vi "FipsAdjacent.vi"() -> (11 "Fips":i32[](array[numeric]))   [LabVIEW 2017] (continued)
41067\t\"Tillamook County, OR\"\t41057\n\"Washington County, OR\"\t41067\t\"Washington County, OR\"\t41067\n\"Washington County, OR\"\t41067\t\"Yamhill County, OR\"\t41071\n\"Wheeler County, OR\"\t41069\t\"Crook County, OR\"\t41013\n\"Wheeler County, OR\"\t41069\t\"Gilliam County, OR\"\t41021\n\"Wheeler County, OR\"\t41069\t\"Grant County, OR\"\t41023\n\"Wheeler County, OR\"\t41069\t\"Jefferson County, OR\"\t41031\n\"Wheeler County, OR\"\t41069\t\"Morrow County, OR\"\t41049\n\"Wheeler County, OR\"\t41069\t\"Wasco County, OR\"\t41065\n\"Wheeler County, OR\"\t41069\t\"Wheeler County, OR\"\t41069\n\"Yamhill County, OR\"\t41071\t\"Clackamas County, OR\"\t41005\n\"Yamhill County, OR\"\t41071\t\"Marion County, OR\"\t41047\n\"Yamhill County, OR\"\t41071\t\"Polk County, OR\"\t41053\n\"Yamhill County, OR\"\t41071\t\"Tillamook County, OR\"\t41057\n\"Yamhill County, OR\"\t41071\t\"Washington County, OR\"\t41067\n\"Yamhill County, OR\"\t41071\t\"Yamhill County, OR\"\t41071\n\"Adams County, PA\"\t42001\t\"Carroll County, MD\"\t24013\n\"Adams County, PA\"\t42001\t\"Frederick County, MD\"\t24021\n\"Adams County, PA\"\t42001\t\"Adams County, PA\"\t42001\n\"Adams County, PA\"\t42001\t\"Cumberland County, PA\"\t42041\n\"Adams County, PA\"\t42001\t\"Franklin County, PA\"\t42055\n\"Adams County, PA\"\t42001\t\"York County, PA\"\t42133\n\"Allegheny County, PA\"\t42003\t\"Allegheny County, PA\"\t42003\n\"Allegheny County, PA\"\t42003\t\"Armstrong County, PA\"\t42005\n\"Allegheny County, PA\"\t42003\t\"Beaver County, PA\"\t42007\n\"Allegheny County, PA\"\t42003\t\"Butler County, PA\"\t42019\n\"Allegheny County, PA\"\t42003\t\"Washington County, PA\"\t42125\n\"Allegheny County, PA\"\t42003\t\"Westmoreland County, PA\"\t42129\n\"Armstrong County, PA\"\t42005\t\"Allegheny County, PA\"\t42003\n\"Armstrong County, PA\"\t42005\t\"Armstrong County, PA\"\t42005\n\"Armstrong County, PA\"\t42005\t\"Butler County, PA\"\t42019\n\"Armstrong County, PA\"\t42005\t\"Clarion County, PA\"\t42031\n\"Armstrong County, PA\"\t42005\t\"Indiana County, PA\"\t42063\n\"Armstrong County, PA\"\t42005\t\"Jefferson County, PA\"\t42065\n\"Armstrong County, PA\"\t42005\t\"Westmoreland County, PA\"\t42129\n\"Beaver County, PA\"\t42007\t\"Columbiana County, OH\"\t39029\n\"Beaver County, PA\"\t42007\t\"Allegheny County, PA\"\t42003\n\"Beaver County, PA\"\t42007\t\"Beaver County, PA\"\t42007\n\"Beaver County, PA\"\t42007\t\"Butler County, PA\"\t42019\n\"Beaver County, PA\"\t42007\t\"Lawrence County, PA\"\t42073\n\"Beaver County, PA\"\t42007\t\"Washington County, PA\"\t42125\n\"Beaver County, PA\"\t42007\t\"Hancock County, WV\"\t54029\n\"Bedford County, PA\"\t42009\t\"Allegany County, MD\"\t24001\n\"Bedford County, PA\"\t42009\t\"Bedford County, PA\"\t42009\n\"Bedford County, PA\"\t42009\t\"Blair County, PA\"\t42013\n\"Bedford County, PA\"\t42009\t\"Cambria County, PA\"\t42021\n\"Bedford County, PA\"\t42009\t\"Fulton County, PA\"\t42057\n\"Bedford County, PA\"\t42009\t\"Huntingdon County, PA\"\t42061\n\"Bedford County, PA\"\t42009\t\"Somerset County, PA\"\t42111\n\"Berks County, PA\"\t42011\t\"Berks County, PA\"\t42011\n\"Berks County, PA\"\t42011\t\"Chester County, PA\"\t42029\n\"Berks County, PA\"\t42011\t\"Lancaster County, PA\"\t42071\n\"Berks County, PA\"\t42011\t\"Lebanon County, PA\"\t42075\n\"Berks County, PA\"\t42011\t\"Lehigh County, PA\"\t42077\n\"Berks County, PA\"\t42011\t\"Montgomery County, PA\"\t42091\n\"Berks County, PA\"\t42011\t\"Schuylkill County, PA\"\t42107\n\"Blair County, PA\"\t42013\t\"Bedford County, PA\"\t42009\n\"Blair County, PA\"\t42013\t\"Blair County, PA\"\t42013\n\"Blair County, PA\"\t42013\t\"Cambria County, PA\"\t42021\n\"Blair County, PA\"\t42013\t\"Centre County, PA\"\t42027\n\"Blair County, PA\"\t42013\t\"Clearfield County, PA\"\t42033\n\"Blair County, PA\"\t42013\t\"Huntingdon County, PA\"\t42061\n\"Bradford County, PA\"\t42015\t\"Chemung County, NY\"\t36015\n\"Bradford County, PA\"\t42015\t\"Tioga County, NY\"\t36107\n\"Bradford County, PA\"\t42015\t\"Bradford County, PA\"\t42015\n\"Bradford County, PA\"\t42015\t\"Lycoming County, PA\"\t42081\n\"Bradford County, PA\"\t42015\t\"Sullivan County, PA\"\t42113\n\"Bradford County, PA\"\t42015\t\"Susquehanna County, PA\"\t42115\n\"Bradford County, PA\"\t42015\t\"Tioga County, PA\"\t42117\n\"Bradford County, PA\"\t42015\t\"Wyoming County, PA\"\t42131\n\"Bucks County, PA\"\t42017\t\"Burlington County, NJ\"\t34005\n\"Bucks County, PA\"\t42017\t\"Hunterdon County, NJ\"\t34019\n\"Bucks County, PA\"\t42017\t\"Mercer County, NJ\"\t34021\n\"Bucks County, PA\"\t42017\t\"Warren County, NJ\"\t34041\n\"Bucks County, PA\"\t42017\t\"Bucks County, PA\"\t42017\n\"Bucks County, PA\"\t42017\t\"Lehigh County, PA\"\t42077\n\"Bucks County, PA\"\t42017\t\"Montgomery County, PA\"\t42091\n\"Bucks County, PA\"\t42017\t\"Northampton County, PA\"\t42095\n\"Bucks County, PA\"\t42017\t\"Philadelphia County, PA\"\t42101\n\"Butler County, PA\"\t42019\t\"Allegheny County, PA\"\t42003\n\"Butler County, PA\"\t42019\t\"Armstrong County, PA\"\t42005\n\"Butler County, PA\"\t42019\t\"Beaver County, PA\"\t42007\n\"Butler County, PA\"\t42019\t\"Butler County, PA\"\t42019\n\"Butler County, PA\"\t42019\t\"Clarion County, PA\"\t42031\n\"Butler County, PA\"\t42019\t\"Lawrence County, PA\"\t42073\n\"Butler County, PA\"\t42019\t\"Mercer County, PA\"\t42085\n\"Butler County, PA\"\t42019\t\"Venango County, PA\"\t42121\n\"Cambria County, PA\"\t42021\t\"Bedford County, PA\"\t42009\n\"Cambria County, PA\"\t42021\t\"Blair County, PA\"\t42013\n\"Cambria County, PA\"\t42021\t\"Cambria County, PA\"\t42021\n\"Cambria County, PA\"\t42021\t\"Clearfield County, PA\"\t42033\n\"Cambria County, PA\"\t42021\t\"Indiana County, PA\"\t42063\n\"Cambria County, PA\"\t42021\t\"Somerset County, PA\"\t42111\n\"Cambria County, PA\"\t42021\t\"Westmoreland County, PA\"\t42129\n\"Cameron County, PA\"\t42023\t\"Cameron County, PA\"\t42023\n\"Cameron County, PA\"\t42023\t\"Clearfield County, PA\"\t42033\n\"Cameron County, PA\"\t42023\t\"Clinton County, PA\"\t42035\n\"Cameron County, PA\"\t42023\t\"Elk County, PA\"\t42047\n\"Cameron County, PA\"\t42023\t\"McKean County, PA\"\t42083\n\"Cameron County, PA\"\t42023\t\"Potter County, PA\"\t42105\n\"Carbon County, PA\"\t42025\t\"Carbon County, PA\"\t42025\n\"Carbon County, PA\"\t42025\t\"Lehigh County, PA\"\t42077\n\"Carbon County, PA\"\t42025\t\"Luzerne County, PA\"\t42079\n\"Carbon County, PA\"\t42025\t\"Monroe County, PA\"\t42089\n\"Carbon County, PA\"\t42025\t\"Northampton County, PA\"\t42095\n\"Carbon County, PA\"\t42025\t\"Schuylkill County, PA\"\t42107\n\"Centre County, PA\"\t42027\t\"Blair County, PA\"\t42013\n\"Centre County, PA\"\t42027\t\"Centre County, PA\"\t42027\n\"Centre County, PA\"\t42027\t\"Clearfield County, PA\"\t42033\n\"Centre County, PA\"\t42027\t\"Clinton County, PA\"\t42035\n\"Centre County, PA\"\t42027\t\"Huntingdon County, PA\"\t42061\n\"Centre County, PA\"\t42027\t\"Mifflin County, PA\"\t42087\n\"Centre County, PA\"\t42027\t\"Union County, PA\"\t42119\n\"Chester County, PA\"\t42029\t\"New Castle County, DE\"\t10003\n\"Chester County, PA\"\t42029\t\"Cecil County, MD\"\t24015\n\"Chester County, PA\"\t42029\t\"Berks County, PA\"\t42011\n\"Chester County, PA\"\t42029\t\"Chester County, PA\"\t42029\n\"Chester County, PA\"\t42029\t\"Delaware County, PA\"\t42045\n\"Chester County, PA\"\t42029\t\"Lancaster County, PA\"\t42071\n\"Chester County, PA\"\t42029\t\"Montgomery County, PA\"\t42091\n\"Clarion County, PA\"\t42031\t\"Armstrong County, PA\"\t42005\n\"Clarion County, PA\"\t42031\t\"Butler County, PA\"\t42019\n\"Clarion County, PA\"\t42031\t\"Clarion County, PA\"\t42031\n\"Clarion County, PA\"\t42031\t\"Forest County, PA\"\t42053\n\"Clarion County, PA\"\t42031\t\"Jefferson County, PA\"\t42065\n\"Clarion County, PA\"\t42031\t\"Venango County, PA\"\t42121\n\"Clearfield County, PA\"\t42033\t\"Blair County, PA\"\t42013\n\"Clearfield County, PA\"\t42033\t\"Cambria County, PA\"\t42021\n\"Clearfield County, PA\"\t42033\t\"Cameron County, PA\"\t42023\n\"Clearfield County, PA\"\t42033\t\"Centre County, PA\"\t42027\n\"Clearfield County, PA\"\t42033\t\"Clearfield County, PA\"\t42033\n\"Clearfield County, PA\"\t42033\t\"Clinton County, PA\"\t42035\n\"Clearfield County, PA\"\t42033\t\"Elk County, PA\"\t42047\n\"Clearfield County, PA\"\t42033\t\"Indiana County, PA\"\t42063\n\"Clearfield County, PA\"\t42033\t\"Jefferson County, PA\"\t42065\n\"Clinton County, PA\"\t42035\t\"Cameron County, PA\"\t42023\n\"Clinton County, PA\"\t42035\t\"Centre County, PA\"\t42027\n\"Clinton County, PA\"\t42035\t\"Clearfield County, PA\"\t42033\n\"Clinton County, PA\"\t42035\t\"Clinton County, PA\"\t42035\n\"Clinton County, PA\"\t42035\t\"Lycoming County, PA\"\t42081\n\"Clinton County, PA\"\t42035\t\"Potter County, PA\"\t42105\n\"Clinton County, PA\"\t42035\t\"Union County, PA\"\t42119\n\"Columbia County, PA\"\t42037\t\"Columbia County, PA\"\t42037\n\"Columbia County, PA\"\t42037\t\"Luzerne County, PA\"\t42079\n\"Columbia County, PA\"\t42037\t\"Lycoming County, PA\"\t42081\n\"Columbia County, PA\"\t42037\t\"Montour County, PA\"\t42093\n\"Columbia County, PA\"\t42037\t\"Northumberland County, PA\"\t42097\n\"Columbia County, PA\"\t42037\t\"Schuylkill County, PA\"\t42107\n\"Columbia County, PA\"\t42037\t\"Sullivan County, PA\"\t42113\n\"Crawford County, PA\"\t42039\t\"Ashtabula County, OH\"\t39007\n\"Crawford County, PA\"\t42039\t\"Trumbull County, OH\"\t39155\n\"Crawford County, PA\"\t42039\t\"Crawford County, PA\"\t42039\n\"Crawford County, PA\"\t42039\t\"Erie County, PA\"\t42049\n\"Crawford County, PA\"\t42039\t\"Mercer County, PA\"\t42085\n\"Crawford County, PA\"\t42039\t\"Venango County, PA\"\t42121\n\"Crawford County, PA\"\t42039\t\"Warren County, PA\"\t42123\n\"Cumberland County, PA\"\t42041\t\"Adams County, PA\"\t42001\n\"Cumberland County, PA\"\t42041\t\"Cumberland County, PA\"\t42041\n\"Cumberland County, PA\"\t42041\t\"Dauphin County, PA\"\t42043\n\"Cumberland County, PA\"\t42041\t\"Franklin County, PA\"\t42055\n\"Cumberland County, PA\"\t42041\t\"Perry County, PA\"\t42099\n\"Cumberland County, PA\"\t42041\t\"York County, PA\"\t42133\n\"Dauphin County, PA\"\t42043\t\"Cumberland County, PA\"\t42041\n\"Dauphin County, PA\"\t42043\t\"Dauphin County, PA\"\t42043\n\"Dauphin County, PA\"\t42043\t\"Juniata County, PA\"\t42067\n\"Dauphin County, PA\"\t42043\t\"Lancaster County, PA\"\t42071\n\"Dauphin County, PA\"\t42043\t\"Lebanon County, PA\"\t42075\n\"Dauphin County, PA\"\t42043\t\"Northumberland County, PA\"\t42097\n\"Dauphin County, PA\"\t42043\t\"Perry County, PA\"\t42099\n\"Dauphin County, PA\"\t42043\t\"Schuylkill County, PA\"\t42107\n\"Dauphin County, PA\"\t42043\t\"York County, PA\"\t42133\n\"Delaware County, PA\"\t42045\t\"New Castle County, DE\"\t10003\n\"Delaware County, PA\"\t42045\t\"Gloucester County, NJ\"\t34015\n\"Delaware County, PA\"\t42045\t\"Chester County, PA\"\t42029\n\"Delaware County, PA\"\t42045\t\"Delaware County, PA\"\t42045\n\"Delaware County, PA\"\t42045\t\"Montgomery County, PA\"\t42091\n\"Delaware County, PA\"\t42045\t\"Philadelphia County, PA\"\t42101\n\"Elk County, PA\"\t42047\t\"Cameron County, PA\"\t42023\n\"Elk County, PA\"\t42047\t\"Clearfield County, PA\"\t42033\n\"Elk County, PA\"\t42047\t\"Elk County, PA\"\t42047\n\"Elk County, PA\"\t42047\t\"Forest County, PA\"\t42053\n\"Elk County, PA\"\t42047\t\"Jefferson County, PA\"\t42065\n\"Elk County, PA\"\t42047\t\"McKean County, PA\"\t42083\n\"Elk County, PA\"\t42047\t\"Warren County, PA\"\t42123\n\"Erie County, PA\"\t42049\t\"Chautauqua County, NY\"\t36013\n\"Erie County, PA\"\t42049\t\"Ashtabula County, OH\"\t39007\n\"Erie County, PA\"\t42049\t\"Crawford County, PA\"\t42039\n\"Erie County, PA\"\t42049\t\"Erie County, PA\"\t42049\n\"Erie County, PA\"\t42049\t\"Warren County, PA\"\t42123\n\"Fayette County, PA\"\t42051\t\"Garrett County, MD\"\t24023\n\"Fayette County, PA\"\t42051\t\"Fayette County, PA\"\t42051\n\"Fayette County, PA\"\t42051\t\"Greene County, PA\"\t42059\n\"Fayette County, PA\"\t42051\t\"Somerset County, PA\"\t42111\n\"Fayette County, PA\"\t42051\t\"Washington County, PA\"\t42125\n\"Fayette County, PA\"\t42051\t\"Westmoreland County, PA\"\t42129\n\"Fayette County, PA\"\t42051\t\"Monongalia County, WV\"\t54061\n\"Fayette County, PA\"\t42051\t\"Preston County, WV\"\t54077\n\"Forest County, PA\"\t42053\t\"Clarion County, PA\"\t42031\n\"Forest County, PA\"\t42053\t\"Elk County, PA\"\t42047\n\"Forest County, PA\"\t42053\t\"Forest County, PA\"\t42053\n\"Forest County, PA\"\t42053\t\"Jefferson County, PA\"\t42065\n\"Forest County, PA\"\t42053\t\"Venango County, PA\"\t42121\n\"Forest County, PA\"\t42053\t\"Warren County, PA\"\t42123\n\"Franklin County, PA\"\t42055\t\"Frederick County, MD\"\t24021\n\"Franklin County, PA\"\t42055\t\"Washington County, MD\"\t24043\n\"Franklin County, PA\"\t42055\t\"Adams County, PA\"\t42001\n\"Franklin County, PA\"\t42055\t\"Cumberland County, PA\"\t42041\n\"Franklin County, PA\"\t42055\t\"Franklin County, PA\"\t42055\n\"Franklin County, PA\"\t42055\t\"Fulton County, PA\"\t42057\n\"Franklin County, PA\"\t42055\t\"Huntingdon County, PA\"\t42061\n\"Franklin County, PA\"\t42055\t\"Juniata County, PA\"\t42067\n\"Franklin County, PA\"\t42055\t\"Perry County, PA\"\t42099\n\"Fulton County, PA\"\t42057\t\"Allegany County, MD\"\t24001\n\"Fulton County, PA\"\t42057\t\"Washington County, MD\"\t24043\n\"Fulton County, PA\"\t42057\t\"Bedford County, PA\"\t42009\n\"Fulton County, PA\"\t42057\t\"Franklin County, PA\"\t42055\n\"Fulton County, PA\"\t42057\t\"Fulton County, PA\"\t42057\n\"Fulton County, PA\"\t42057\t\"Huntingdon County, PA\"\t42061\n\"Greene County, PA\"\t42059\t\"Fayette County, PA\"\t42051\n\"Greene County, PA\"\t42059\t\"Greene County, PA\"\t42059\n\"Greene County, PA\"\t42059\t\"Washington County, PA\"\t42125\n\"Greene County, PA\"\t42059\t\"Marshall County, WV\"\t54051\n\"Greene County, PA\"\t42059\t\"Monongalia County, WV\"\t54061\n\"Greene County, PA\"\t42059\t\"Wetzel County, WV\"\t54103\n\"Huntingdon County, PA\"\t42061\t\"Bedford County, PA\"\t42009\n\"Huntingdon County, PA\"\t42061\t\"Blair County, PA\"\t42013\n\"Huntingdon County, PA\"\t42061\t\"Centre County, PA\"\t42027\n\"Huntingdon County, PA\"\t42061\t\"Franklin County, PA\"\t42055\n\"Huntingdon County, PA\"\t42061\t\"Fulton County, PA\"\t42057\n\"Huntingdon County, PA\"\t42061\t\"Huntingdon County, PA\"\t42061\n\"Huntingdon County, PA\"\t42061\t\"Juniata County, PA\"\t42067\n\"Huntingdon County, PA\"\t42061\t\"Mifflin County, PA\"\t42087\n\"Indiana County, PA\"\t42063\t\"Armstrong County, PA\"\t42005\n\"Indiana County, PA\"\t42063\t\"Cambria County, PA\"\t42021\n\"Indiana County, PA\"\t42063\t\"Clearfield County, PA\"\t42033\n\"Indiana County, PA\"\t42063\t\"Indiana County, PA\"\t42063\n\"Indiana County, PA\"\t42063\t\"Jefferson County, PA\"\t42065\n\"Indiana County, PA\"\t42063\t\"Westmoreland County, PA\"\t42129\n\"Jefferson County, PA\"\t42065\t\"Armstrong County, PA\"\t42005\n\"Jefferson County, PA\"\t42065\t\"Clarion County, PA\"\t42031\n\"Jefferson County, PA\"\t42065\t\"Clearfield County, PA\"\t42033\n\"Jefferson County, PA\"\t42065\t\"Elk County, PA\"\t42047\n\"Jefferson County, PA\"\t42065\t\"Forest County, PA\"\t42053\n\"Jefferson County, PA\"\t42065\t\"Indiana County, PA\"\t42063\n\"Jefferson County, PA\"\t42065\t\"Jefferson County, PA\"\t42065\n\"Juniata County, PA\"\t42067\t\"Dauphin County, PA\"\t42043\n\"Juniata County, PA\"\t42067\t\"Franklin County, PA\"\t42055\n\"Juniata County, PA\"\t42067\t\"Huntingdon County, PA\"\t42061\n\"Juniata County, PA\"\t42067\t\"Juniata County, PA\"\t42067\n\"Juniata County, PA\"\t42067\t\"Mifflin County, PA\"\t42087\n\"Juniata County, PA\"\t42067\t\"Northumberland County, PA\"\t42097\n\"Juniata County, PA\"\t42067\t\"Perry County, PA\"\t42099\n\"Juniata County, PA\"\t42067\t\"Snyder County, PA\"\t42109\n\"Lackawanna County, PA\"\t42069\t\"Lackawanna County, PA\"\t42069\n\"Lackawanna County, PA\"\t42069\t\"Luzerne County, PA\"\t42079\n\"Lackawanna County, PA\"\t42069\t\"Monroe County, PA\"\t42089\n\"Lackawanna County, PA\"\t42069\t\"Susquehanna County, PA\"\t42115\n\"Lackawanna County, PA\"\t42069\t\"Wayne County, PA\"\t42127\n\"Lackawanna County, PA\"\t42069\t\"Wyoming County, PA\"\t42131\n\"Lancaster County, PA\"\t42071\t\"Cecil County, MD\"\t24015\n\"Lancaster County, PA\"\t42071\t\"Harford County, MD\"\t24025\n\"Lancaster County, PA\"\t42071\t\"Berks County, PA\"\t42011\n\"Lancaster County, PA\"\t42071\t\"Chester County, PA\"\t42029\n\"Lancaster County, PA\"\t42071\t\"Dauphin County, PA\"\t42043\n\"Lancaster County, PA\"\t42071\t\"Lancaster County, PA\"\t42071\n\"Lancaster County, PA\"\t42071\t\"Lebanon County, PA\"\t42075\n\"Lancaster County, PA\"\t42071\t\"York County, PA\"\t42133\n\"Lawrence County, PA\"\t42073\t\"Columbiana County, OH\"\t39029\n\"Lawrence County, PA\"\t42073\t\"Mahoning County, OH\"\t39099\n\"Lawrence County, PA\"\t42073\t\"Beaver County, PA\"\t42007\n\"Lawrence County, PA\"\t42073\t\"Butler County, PA\"\t42019\n\"Lawrence County, PA\"\t42073\t\"Lawrence County, PA\"\t42073\n\"Lawrence County, PA\"\t42073\t\"Mercer County, PA\"\t42085\n\"Lebanon County, PA\"\t42075\t\"Berks County, PA\"\t42011\n\"Lebanon County, PA\"\t42075\t\"Dauphin County, PA\"\t42043\n\"Lebanon County, PA\"\t42075\t\"Lancaster County, PA\"\t42071\n\"Lebanon County, PA\"\t42075\t\"Lebanon County, PA\"\t42075\n\"Lebanon County, PA\"\t42075\t\"Schuylkill County, PA\"\t42107\n\"Lehigh County, PA\"\t42077\t\"Berks County, PA\"\t42011\n\"Lehigh County, PA\"\t42077\t\"Bucks County, PA\"\t42017\n\"Lehigh County, PA\"\t42077\t\"Carbon County, PA\"\t42025\n\"Lehigh County, PA\"\t42077\t\"Lehigh County, PA\"\t42077\n\"Lehigh County, PA\"\t42077\t\"Montgomery County, PA\"\t42091\n\"Lehigh County, PA\"\t42077\t\"Northampton County, PA\"\t42095\n\"Lehigh County, PA\"\t42077\t\"Schuylkill County, PA\"\t42107\n\"Luzerne County, PA\"\t42079\t\"Carbon County, PA\"\t42025\n\"Luzerne County, PA\"\t42079\t\"Columbia County, PA\"\t42037\n\"Luzerne County, PA\"\t42079\t\"Lackawanna County, PA\"\t42069\n\"Luzerne County, PA\"\t42079\t\"Luzerne County, PA\"\t42079\n\"Luzerne County, PA\"\t42079\t\"Monroe County, PA\"\t42089\n\"Luzerne County, PA\"\t42079\t\"Schuylkill County, PA\"\t42107\n\"Luzerne County, PA\"\t42079\t\"Sullivan County, PA\"\t42113\n\"Luzerne County, PA\"\t42079\t\"Wyoming County, PA\"\t42131\n\"Lycoming County, PA\"\t42081\t\"Bradford County, PA\"\t42015\n\"Lycoming County, PA\"\t42081\t\"Clinton County, PA\"\t42035\n\"Lycoming County, PA\"\t42081\t\"Columbia County, PA\"\t42037\n\"Lycoming County, PA\"\t42081\t\"Lycoming County, PA\"\t42081\n\"Lycoming County, PA\"\t42081\t\"Montour County, PA\"\t42093\n\"Lycoming County, PA\"\t42081\t\"Northumberland County, PA\"\t42097\n\"Lycoming County, PA\"\t42081\t\"Potter County, PA\"\t42105\n\"Lycoming County, PA\"\t42081\t\"Sullivan County, PA\"\t42113\n\"Lycoming County, PA\"\t42081\t\"Tioga County, PA\"\t42117\n\"Lycoming County, PA\"\t42081\t\"Union County, PA\"\t42119\n\"McKean County, PA\"\t42083\t\"Allegany County, NY\"\t36003\n\"McKean County, PA\"\t42083\t\"Cattaraugus County, NY\"\t36009\n\"McKean County, PA\"\t42083\t\"Cameron County, PA\"\t42023\n\"McKean County, PA\"\t42083\t\"Elk County, PA\"\t42047\n\"McKean County, PA\"\t42083\t\"McKean County, PA\"\t42083\n\"McKean County, PA\"\t42083\t\"Potter County, PA\"\t42105\n\"McKean County, PA\"\t42083\t\"Warren County, PA\"\t42123\n\"Mercer County, PA\"\t42085\t\"Mahoning County, OH\"\t39099\n\"Mercer County, PA\"\t42085\t\"Trumbull County, OH\"\t39155\n\"Mercer County, PA\"\t42085\t\"Butler County, PA\"\t42019\n\"Mercer County, PA\"\t42085\t\"Crawford County, PA\"\t42039\n\"Mercer County, PA\"\t42085\t\"Lawrence County, PA\"\t42073\n\"Mercer County, PA\"\t42085\t\"Mercer County, PA\"\t42085\n\"Mercer County, PA\"\t42085\t\"Venango County, PA\"\t42121\n\"Mifflin County, PA\"\t42087\t\"Centre County, PA\"\t42027\n\"Mifflin County, PA\"\t42087\t\"Huntingdon County, PA\"\t42061\n\"Mifflin County, PA\"\t42087\t\"Juniata County, PA\"\t42067\n\"Mifflin County, PA\"\t42087\t\"Mifflin County, PA\"\t42087\n\"Mifflin County, PA\"\t42087\t\"Snyder County, PA\"\t42109\n\"Mifflin County, PA\"\t42087\t\"Union County, PA\"\t42119\n\"Monroe County, PA\"\t42089\t\"Sussex County, NJ\"\t34037\n\"Monroe County, PA\"\t42089\t\"Warren County, NJ\"\t34041\n\"Monroe County, PA\"\t42089\t\"Carbon County, PA\"\t42025\n\"Monroe County, PA\"\t42089\t\"Lackawanna County, PA\"\t42069\n\"Monroe County, PA\"\t42089\t\"Luzerne County, PA\"\t42079\n\"Monroe County, PA\"\t42089\t\"Monroe County, PA\"\t42089\n\"Monroe County, PA\"\t42089\t\"Northampton County, PA\"\t42095\n\"Monroe County, PA\"\t42089\t\"Pike County, PA\"\t42103\n\"Monroe County, PA\"\t42089\t\"Wayne County, PA\"\t42127\n\"Montgomery County, PA\"\t42091\t\"Berks County, PA\"\t42011\n\"Montgomery County, PA\"\t42091\t\"Bucks County, PA\"\t42017\n\"Montgomery County, PA\"\t42091\t\"Chester County, PA\"\t42029\n\"Montgomery County, PA\"\t42091\t\"Delaware County, PA\"\t42045\n\"Montgomery County, PA\"\t42091\t\"Lehigh County, PA\"\t42077\n\"Montgomery County, PA\"\t42091\t\"Montgomery County, PA\"\t42091\n\"Montgomery County, PA\"\t42091\t\"Philadelphia County, PA\"\t42101\n\"Montour County, PA\"\t42093\t\"Columbia County, PA\"\t42037\n\"Montour County, PA\"\t42093\t\"Lycoming County, PA\"\t42081\n\"Montour County, PA\"\t42093\t\"Montour County, PA\"\t42093\n\"Montour County, PA\"\t42093\t\"Northumberland County, PA\"\t42097\n\"Northampton County, PA\"\t42095\t\"Warren County, NJ\"\t34041\n\"Northampton County, PA\"\t42095\t\"Bucks County, PA\"\t42017\n\"Northampton County, PA\"\t42095\t\"Carbon County, PA\"\t42025\n\"Northampton County, PA\"\t42095\t\"Lehigh County, PA\"\t42077\n\"Northampton County, PA\"\t42095\t\"Monroe County, PA\"\t42089\n\"Northampton County, PA\"\t42095\t\"Northampton County, PA\"\t42095\n\"Northumberland County, PA\"\t42097\t\"Columbia County, PA\"\t42037\n\"Northumberland County, PA\"\t42097\t\"Dauphin County, PA\"\t42043\n\"Northumberland County, PA\"\t42097\t\"Juniata County, PA\"\t42067\n\"Northumberland County, PA\"\t42097\t\"Lycoming County, PA\"\t42081\n\"Northumberland County, PA\"\t42097\t\"Montour County, PA\"\t42093\n\"Northumberland County, PA\"\t42097\t\"Northumberland County, PA\"\t42097\n\"Northumberland County, PA\"\t42097\t\"Perry County, PA\"\t42099\n\"Northumberland County, PA\"\t42097\t\"Schuylkill County, PA\"\t42107\n\"Northumberland County, PA\"\t42097\t\"Snyder County, PA\"\t42109\n\"Northumberland County, PA\"\t42097\t\"Union County, PA\"\t42119\n\"Perry County, PA\"\t42099\t\"Cumberland County, PA\"\t42041\n\"Perry County, PA\"\t42099\t\"Dauphin County, PA\"\t42043\n\"Perry County, PA\"\t42099\t\"Franklin County, PA\"\t42055\n\"Perry County, PA\"\t42099\t\"Juniata County, PA\"\t42067\n\"Perry County, PA\"\t42099\t\"Northumberland County, PA\"\t42097\n\"Perry County, PA\"\t42099\t\"Perry County, PA\"\t42099\n\"Philadelphia County, PA\"\t42101\t\"Burlington County, NJ\"\t34005\n\"Philadelphia County, PA\"\t42101\t\"Camden County, NJ\"\t34007\n\"Philadelphia County, PA\"\t42101\t\"Gloucester County, NJ\"\t34015\n\"Philadelphia County, PA\"\t42101\t\"Bucks County, PA\"\t42017\n\"Philadelphia County, PA\"\t42101\t\"Delaware County, PA\"\t42045\n\"Philadelphia County, PA\"\t42101\t\"Montgomery County, PA\"\t42091\n\"Philadelphia County, PA\"\t42101\t\"Philadelphia County, PA\"\t42101\n\"Pike County, PA\"\t42103\t\"Sussex County, NJ\"\t34037\n\"Pike County, PA\"\t42103\t\"Orange County, NY\"\t36071\n\"Pike County, PA\"\t42103\t\"Sullivan County, NY\"\t36105\n\"Pike County, PA\"\t42103\t\"Monroe County, PA\"\t42089\n\"Pike County, PA\"\t42103\t\"Pike County, PA\"\t42103\n\"Pike County, PA\"\t42103\t\"Wayne County, PA\"\t42127\n\"Potter County, PA\"\t42105\t\"Allegany County, NY\"\t36003\n\"Potter County, PA\"\t42105\t\"Steuben County, NY\"\t36101\n\"Potter County, PA\"\t42105\t\"Cameron County, PA\"\t42023\n\"Potter County, PA\"\t42105\t\"Clinton County, PA\"\t42035\n\"Potter County, PA\"\t42105\t\"Lycoming County, PA\"\t42081\n\"Potter County, PA\"\t42105\t\"McKean County, PA\"\t42083\n\"Potter County, PA\"\t42105\t\"Potter County, PA\"\t42105\n\"Potter County, PA\"\t42105\t\"Tioga County, PA\"\t42117\n\"Schuylkill County, PA\"\t42107\t\"Berks County, PA\"\t42011\n\"Schuylkill County, PA\"\t42107\t\"Carbon County, PA\"\t42025\n\"Schuylkill County, PA\"\t42107\t\"Columbia County, PA\"\t42037\n\"Schuylkill County, PA\"\t42107\t\"Dauphin County, PA\"\t42043\n\"Schuylkill County, PA\"\t42107\t\"Lebanon County, PA\"\t42075\n\"Schuylkill County, PA\"\t42107\t\"Lehigh County, PA\"\t42077\n\"Schuylkill County, PA\"\t42107\t\"Luzerne County, PA\"\t42079\n\"Schuylkill County, PA\"\t42107\t\"Northumberland County, PA\"\t42097\n\"Schuylkill County, PA\"\t42107\t\"Schuylkill County, PA\"\t42107\n\"Snyder County, PA\"\t42109\t\"Juniata County, PA\"\t42067\n\"Snyder County, PA\"\t42109\t\"Mifflin County, PA\"\t42087\n\"Snyder County, PA\"\t42109\t\"Northumberland County, PA\"\t42097\n\"Snyder County, PA\"\t42109\t\"Snyder County, PA\"\t42109\n\"Snyder County, PA\"\t42109\t\"Union County, PA\"\t42119\n\"Somerset County, PA\"\t42111\t\"Allegany County, MD\"\t24001\n\"Somerset County, PA\"\t42111\t\"Garrett County, MD\"\t24023\n\"Somerset County, PA\"\t42111\t\"Bedford County, PA\"\t42009\n\"Somerset County, PA\"\t42111\t\"Cambria County, PA\"\t42021\n\"Somerset County, PA\"\t42111\t\"Fayette County, PA\"\t42051\n\"Somerset County, PA\"\t42111\t\"Somerset County, PA\"\t42111\n\"Somerset County, PA\"\t42111\t\"Westmoreland County, PA\"\t42129\n\"Sullivan County, PA\"\t42113\t\"Bradford County, PA\"\t42015\n\"Sullivan County, PA\"\t42113\t\"Columbia County, PA\"\t42037\n\"Sullivan County, PA\"\t42113\t\"Luzerne County, PA\"\t42079\n\"Sullivan County, PA\"\t42113\t\"Lycoming County, PA\"\t42081\n\"Sullivan County, PA\"\t42113\t\"Sullivan County, PA\"\t42113\n\"Sullivan County, PA\"\t42113\t\"Wyoming County, PA\"\t42131\n\"Susquehanna County, PA\"\t42115\t\"Broome County, NY\"\t36007\n\"Susquehanna County, PA\"\t42115\t\"Tioga County, NY\"\t36107\n\"Susquehanna County, PA\"\t42115\t\"Bradford County, PA\"\t42015\n\"Susquehanna County, PA\"\t42115\t\"Lackawanna County, PA\"\t42069\n\"Susquehanna County, PA\"\t42115\t\"Susquehanna County, PA\"\t42115\n\"Susquehanna County, PA\"\t42115\t\"Wayne County, PA\"\t42127\n\"Susquehanna County, PA\"\t42115\t\"Wyoming County, PA\"\t42131\n\"Tioga County, PA\"\t42117\t\"Chemung County, NY\"\t36015\n\"Tioga County, PA\"\t42117\t\"Steuben County, NY\"\t36101\n\"Tioga County, PA\"\t42117\t\"Bradford County, PA\"\t42015\n\"Tioga County, PA\"\t42117\t\"Lycoming County, PA\"\t42081\n\"Tioga County, PA\"\t42117\t\"Potter County, PA\"\t42105\n\"Tioga County, PA\"\t42117\t\"Tioga County, PA\"\t42117\n\"Union County, PA\"\t42119\t\"Centre County, PA\"\t42027\n\"Union County, PA\"\t42119\t\"Clinton County, PA\"\t42035\n\"Union County, PA\"\t42119\t\"Lycoming County, PA\"\t42081\n\"Union County, PA\"\t42119\t\"Mifflin County, PA\"\t42087\n\"Union County, PA\"\t42119\t\"Northumberland County, PA\"\t42097\n\"Union County, PA\"\t42119\t\"Snyder County, PA\"\t42109\n\"Union County, PA\"\t42119\t\"Union County, PA\"\t42119\n\"Venango County, PA\"\t42121\t\"Butler County, PA\"\t42019\n\"Venango County, PA\"\t42121\t\"Clarion County, PA\"\t42031\n\"Venango County, PA\"\t42121\t\"Crawford County, PA\"\t42039\n\"Venango County, PA\"\t42121\t\"Forest County, PA\"\t42053\n\"Venango County, PA\"\t42121\t\"Mercer County, PA\"\t42085\n\"Venango County, PA\"\t42121\t\"Venango County, PA\"\t42121\n\"Venango County, PA\"\t42121\t\"Warren County, PA\"\t42123\n\"Warren County, PA\"\t42123\t\"Cattaraugus County, NY\"\t36009\n\"Warren County, PA\"\t42123\t\"Chautauqua County, NY\"\t36013\n\"Warren County, PA\"\t42123\t\"Crawford County, PA\"\t42039\n\"Warren County, PA\"\t42123\t\"Elk County, PA\"\t42047\n\"Warren County, PA\"\t42123\t\"Erie County, PA\"\t42049\n\"Warren County, PA\"\t42123\t\"Forest County, PA\"\t42053\n\"Warren County, PA\"\t42123\t\"McKean County, PA\"\t42083\n\"Warren County, PA\"\t42123\t\"Venango County, PA\"\t42121\n\"Warren County, PA\"\t42123\t\"Warren County, PA\"\t42123\n\"Washington County, PA\"\t42125\t\"Allegheny County, PA\"\t42003\n\"Washington County, PA\"\t42125\t\"Beaver County, PA\"\t42007\n\"Washington County, PA\"\t42125\t\"Fayette County, PA\"\t42051\n\"Washington County, PA\"\t42125\t\"Greene County, PA\"\t42059\n\"Washington County, PA\"\t42125\t\"Washington County, PA\"\t42125\n\"Washington County, PA\"\t42125\t\"Westmoreland County, PA\"\t42129\n\"Washington County, PA\"\t42125\t\"Brooke County, WV\"\t54009\n\"Washington County, PA\"\t42125\t\"Hancock County, WV\"\t54029\n\"Washington County, PA\"\t42125\t\"Marshall County, WV\"\t54051\n\"Washington County, PA\"\t42125\t\"Ohio County, WV\"\t54069\n\"Wayne County, PA\"\t42127\t\"Broome County, NY\"\t36007\n\"Wayne County, PA\"\t42127\t\"Delaware County, NY\"\t36025\n\"Wayne County, PA\"\t42127\t\"Sullivan County, NY\"\t36105\n\"Wayne County, PA\"\t42127\t\"Lackawanna County, PA\"\t42069\n\"Wayne County, PA\"\t42127\t\"Monroe County, PA\"\t42089\n\"Wayne County, PA\"\t42127\t\"Pike County, PA\"\t42103\n\"Wayne County, PA\"\t42127\t\"Susquehanna County, PA\"\t42115\n\"Wayne County, PA\"\t42127\t\"Wayne County, PA\"\t42127\n\"Westmoreland County, PA\"\t42129\t\"Allegheny County, PA\"\t42003\n\"Westmoreland County, PA\"\t42129\t\"Armstrong County, PA\"\t42005\n\"Westmoreland County, PA\"\t42129\t\"Cambria County, PA\"\t42021\n\"Westmoreland County, PA\"\t42129\t\"Fayette County, PA\"\t42051\n\"Westmoreland County, PA\"\t42129\t\"Indiana County, PA\"\t42063\n\"Westmoreland County, PA\"\t42129\t\"Somerset County, PA\"\t42111\n\"Westmoreland County, PA\"\t42129\t\"Washington County, PA\"\t42125\n\"Westmoreland County, PA\"\t42129\t\"Westmoreland County, PA\"\t42129\n\"Wyoming County, PA\"\t42131\t\"Bradford County, PA\"\t42015\n\"Wyoming County, PA\"\t42131\t\"Lackawanna County, PA\"\t42069\n\"Wyoming County, PA\"\t42131\t\"Luzerne County, PA\"\t42079\n\"Wyoming County, PA\"\t42131\t\"Sullivan County, PA\"\t42113\n\"Wyoming County, PA\"\t42131\t\"Susquehanna County, PA\"\t42115\n\"Wyoming County, PA\"\t42131\t\"Wyoming County, PA\"\t42131\n\"York County, PA\"\t42133\t\"Baltimore County, MD\"\t24005\n\"York County, PA\"\t42133\t\"Carroll County, MD\"\t24013\n\"York County, PA\"\t42133\t\"Harford County, MD\"\t24025\n\"York County, PA\"\t42133\t\"Adams County, PA\"\t42001\n\"York County, PA\"\t42133\t\"Cumberland County, PA\"\t42041\n\"York County, PA\"\t42133\t\"Dauphin County, PA\"\t42043\n\"York County, PA\"\t42133\t\"Lancaster County, PA\"\t42071\n\"York County, PA\"\t42133\t\"York County, PA\"\t42133\n\"Bristol County, RI\"\t44001\t\"Bristol County, MA\"\t25005\n\"Bristol County, RI\"\t44001\t\"Bristol County, RI\"\t44001\n\"Bristol County, RI\"\t44001\t\"Kent County, RI\"\t44003\n\"Bristol County, RI\"\t44001\t\"Newport County, RI\"\t44005\n\"Bristol County, RI\"\t44001\t\"Providence County, RI\"\t44007\n\"Kent County, RI\"\t44003\t\"New London County, CT\"\t09011\n\"Kent County, RI\"\t44003\t\"Windham County, CT\"\t09015\n\"Kent County, RI\"\t44003\t\"Bristol County, RI\"\t44001\n\"Kent County, RI\"\t44003\t\"Kent County, RI\"\t44003\n\"Kent County, RI\"\t44003\t\"Newport County, RI\"\t44005\n\"Kent County, RI\"\t44003\t\"Providence County, RI\"\t44007\n\"Kent County, RI\"\t44003\t\"Washington County, RI\"\t44009\n\"Newport County, RI\"\t44005\t\"Bristol County, MA\"\t25005\n\"Newport County, RI\"\t44005\t\"Bristol County, RI\"\t44001\n\"Newport County, RI\"\t44005\t\"Kent County, RI\"\t44003\n\"Newport County, RI\"\t44005\t\"Newport County, RI\"\t44005\n\"Newport County, RI\"\t44005\t\"Washington County, RI\"\t44009\n\"Providence County, RI\"\t44007\t\"Windham County, CT\"\t09015\n\"Providence County, RI\"\t44007\t\"Bristol County, MA\"\t25005\n\"Providence County, RI\"\t44007\t\"Norfolk County, MA\"\t25021\n\"Providence County, RI\"\t44007\t\"Worcester County, MA\"\t25027\n\"Providence County, RI\"\t44007\t\"Bristol County, RI\"\t44001\n\"Providence County, RI\"\t44007\t\"Kent County, RI\"\t44003\n\"Providence County, RI\"\t44007\t\"Providence County, RI\"\t44007\n\"Washington County, RI\"\t44009\t\"New London County, CT\"\t09011\n\"Washington County, RI\"\t44009\t\"Suffolk County, NY\"\t36103\n\"Washington County, RI\"\t44009\t\"Kent County, RI\"\t44003\n\"Washington County, RI\"\t44009\t\"Newport County, RI\"\t44005\n\"Washington County, RI\"\t44009\t\"Washington County, RI\"\t44009\n\"Abbeville County, SC\"\t45001\t\"Elbert County, GA\"\t13105\n\"Abbeville County, SC\"\t45001\t\"Abbeville County, SC\"\t45001\n\"Abbeville County, SC\"\t45001\t\"Anderson County, SC\"\t45007\n\"Abbeville County, SC\"\t45001\t\"Greenville County, SC\"\t45045\n\"Abbeville County, SC\"\t45001\t\"Greenwood County, SC\"\t45047\n\"Abbeville County, SC\"\t45001\t\"Laurens County, SC\"\t45059\n\"Abbeville County, SC\"\t45001\t\"McCormick County, SC\"\t45065\n\"Aiken County, SC\"\t45003\t\"Burke County, GA\"\t13033\n\"Aiken County, SC\"\t45003\t\"Richmond County, GA\"\t13245\n\"Aiken County, SC\"\t45003\t\"Aiken County, SC\"\t45003\n\"Aiken County, SC\"\t45003\t\"Barnwell County, SC\"\t45011\n\"Aiken County, SC\"\t45003\t\"Edgefield County, SC\"\t45037\n\"Aiken County, SC\"\t45003\t\"Lexington County, SC\"\t45063\n\"Aiken County, SC\"\t45003\t\"Orangeburg County, SC\"\t45075\n\"Aiken County, SC\"\t45003\t\"Saluda County, SC\"\t45081\n\"Allendale County, SC\"\t45005\t\"Burke County, GA\"\t13033\n\"Allendale County, SC\"\t45005\t\"Screven County, GA\"\t13251\n\"Allendale County, SC\"\t45005\t\"Allendale County, SC\"\t45005\n\"Allendale County, SC\"\t45005\t\"Bamberg County, SC\"\t45009\n\"Allendale County, SC\"\t45005\t\"Barnwell County, SC\"\t45011\n\"Allendale County, SC\"\t45005\t\"Colleton County, SC\"\t45029\n\"Allendale County, SC\"\t45005\t\"Hampton County, SC\"\t45049\n\"Anderson County, SC\"\t45007\t\"Elbert County, GA\"\t13105\n\"Anderson County, SC\"\t45007\t\"Hart County, GA\"\t13147\n\"Anderson County, SC\"\t45007\t\"Abbeville County, SC\"\t45001\n\"Anderson County, SC\"\t45007\t\"Anderson County, SC\"\t45007\n\"Anderson County, SC\"\t45007\t\"Greenville County, SC\"\t45045\n\"Anderson County, SC\"\t45007\t\"Laurens County, SC\"\t45059\n\"Anderson County, SC\"\t45007\t\"Oconee County, SC\"\t45073\n\"Anderson County, SC\"\t45007\t\"Pickens County, SC\"\t45077\n\"Bamberg County, SC\"\t45009\t\"Allendale County, SC\"\t45005\n\"Bamberg County, SC\"\t45009\t\"Bamberg County, SC\"\t45009\n\"Bamberg County, SC\"\t45009\t\"Barnwell County, SC\"\t45011\n\"Bamberg County, SC\"\t45009\t\"Colleton County, SC\"\t45029\n\"Bamberg County, SC\"\t45009\t\"Hampton County, SC\"\t45049\n\"Bamberg County, SC\"\t45009\t\"Orangeburg County, SC\"\t45075\n\"Barnwell County, SC\"\t45011\t\"Burke County, GA\"\t13033\n\"Barnwell County, SC\"\t45011\t\"Aiken County, SC\"\t45003\n\"Barnwell County, SC\"\t45011\t\"Allendale County, SC\"\t45005\n\"Barnwell County, SC\"\t45011\t\"Bamberg County, SC\"\t45009\n\"Barnwell County, SC\"\t45011\t\"Barnwell County, SC\"\t45011\n\"Barnwell County, SC\"\t45011\t\"Orangeburg County, SC\"\t45075\n\"Beaufort County, SC\"\t45013\t\"Beaufort County, SC\"\t45013\n\"Beaufort County, SC\"\t45013\t\"Colleton County, SC\"\t45029\n\"Beaufort County, SC\"\t45013\t\"Hampton County, SC\"\t45049\n\"Beaufort County, SC\"\t45013\t\"Jasper County, SC\"\t45053\n\"Berkeley County, SC\"\t45015\t\"Berkeley County, SC\"\t45015\n\"Berkeley County, SC\"\t45015\t\"Charleston County, SC\"\t45019\n\"Berkeley County, SC\"\t45015\t\"Clarendon County, SC\"\t45027\n\"Berkeley County, SC\"\t45015\t\"Dorchester County, SC\"\t45035\n\"Berkeley County, SC\"\t45015\t\"Georgetown County, SC\"\t45043\n\"Berkeley County, SC\"\t45015\t\"Orangeburg County, SC\"\t45075\n\"Berkeley County, SC\"\t45015\t\"Williamsburg County, SC\"\t45089\n\"Calhoun County, SC\"\t45017\t\"Calhoun County, SC\"\t45017\n\"Calhoun County, SC\"\t45017\t\"Clarendon County, SC\"\t45027\n\"Calhoun County, SC\"\t45017\t\"Lexington County, SC\"\t45063\n\"Calhoun County, SC\"\t45017\t\"Orangeburg County, SC\"\t45075\n\"Calhoun County, SC\"\t45017\t\"Richland County, SC\"\t45079\n\"Calhoun County, SC\"\t45017\t\"Sumter County, SC\"\t45085\n\"Charleston County, SC\"\t45019\t\"Berkeley County, SC\"\t45015\n\"Charleston County, SC\"\t45019\t\"Charleston County, SC\"\t45019\n\"Charleston County, SC\"\t45019\t\"Colleton County, SC\"\t45029\n\"Charleston County, SC\"\t45019\t\"Dorchester County, SC\"\t45035\n\"Charleston County, SC\"\t45019\t\"Georgetown County, SC\"\t45043\n\"Cherokee County, SC\"\t45021\t\"Cleveland County, NC\"\t37045\n\"Cherokee County, SC\"\t45021\t\"Rutherford County, NC\"\t37161\n\"Cherokee County, SC\"\t45021\t\"Cherokee County, SC\"\t45021\n\"Cherokee County, SC\"\t45021\t\"Spartanburg County, SC\"\t45083\n\"Cherokee County, SC\"\t45021\t\"Union County, SC\"\t45087\n\"Cherokee County, SC\"\t45021\t\"York County, SC\"\t45091\n\"Chester County, SC\"\t45023\t\"Chester County, SC\"\t45023\n\"Chester County, SC\"\t45023\t\"Fairfield County, SC\"\t45039\n\"Chester County, SC\"\t45023\t\"Lancaster County, SC\"\t45057\n\"Chester County, SC\"\t45023\t\"Union County, SC\"\t45087\n\"Chester County, SC\"\t45023\t\"York County, SC\"\t45091\n\"Chesterfield County, SC\"\t45025\t\"Anson County, NC\"\t37007\n\"Chesterfield County, SC\"\t45025\t\"Richmond County, NC\"\t37153\n\"Chesterfield County, SC\"\t45025\t\"Union County, NC\"\t37179\n\"Chesterfield County, SC\"\t45025\t\"Chesterfield County, SC\"\t45025\n\"Chesterfield County, SC\"\t45025\t\"Darlington County, SC\"\t45031\n\"Chesterfield County, SC\"\t45025\t\"Kershaw County, SC\"\t45055\n\"Chesterfield County, SC\"\t45025\t\"Lancaster County, SC\"\t45057\n\"Chesterfield County, SC\"\t45025\t\"Marlboro County, SC\"\t45069\n\"Clarendon County, SC\"\t45027\t\"Berkeley County, SC\"\t45015\n\"Clarendon County, SC\"\t45027\t\"Calhoun County, SC\"\t45017\n\"Clarendon County, SC\"\t45027\t\"Clarendon County, SC\"\t45027\n\"Clarendon County, SC\"\t45027\t\"Florence County, SC\"\t45041\n\"Clarendon County, SC\"\t45027\t\"Orangeburg County, SC\"\t45075\n\"Clarendon County, SC\"\t45027\t\"Sumter County, SC\"\t45085\n\"Clarendon County, SC\"\t45027\t\"Williamsburg County, SC\"\t45089\n\"Colleton County, SC\"\t45029\t\"Allendale County, SC\"\t45005\n\"Colleton County, SC\"\t45029\t\"Bamberg County, SC\"\t45009\n\"Colleton County, SC\"\t45029\t\"Beaufort County, SC\"\t45013\n\"Colleton County, SC\"\t45029\t\"Charleston County, SC\"\t45019\n\"Colleton County, SC\"\t45029\t\"Colleton County, SC\"\t45029\n\"Colleton County, SC\"\t45029\t\"Dorchester County, SC\"\t45035\n\"Colleton County, SC\"\t45029\t\"Hampton County, SC\"\t45049\n\"Colleton County, SC\"\t45029\t\"Orangeburg County, SC\"\t45075\n\"Darlington County, SC\"\t45031\t\"Chesterfield County, SC\"\t45025\n\"Darlington County, SC\"\t45031\t\"Darlington County, SC\"\t45031\n\"Darlington County, SC\"\t45031\t\"Florence County, SC\"\t45041\n\"Darlington County, SC\"\t45031\t\"Kershaw County, SC\"\t45055\n\"Darlington County, SC\"\t45031\t\"Lee County, SC\"\t45061\n\"Darlington County, SC\"\t45031\t\"Marlboro County, SC\"\t45069\n\"Dillon County, SC\"\t45033\t\"Columbus County, NC\"\t37047\n\"Dillon County, SC\"\t45033\t\"Robeson County, NC\"\t37155\n\"Dillon County, SC\"\t45033\t\"Dillon County, SC\"\t45033\n\"Dillon County, SC\"\t45033\t\"Florence County, SC\"\t45041\n\"Dillon County, SC\"\t45033\t\"Horry County, SC\"\t45051\n\"Dillon County, SC\"\t45033\t\"Marion County, SC\"\t45067\n\"Dillon County, SC\"\t45033\t\"Marlboro County, SC\"\t45069\n\"Dorchester County, SC\"\t45035\t\"Berkeley County, SC\"\t45015\n\"Dorchester County, SC\"\t45035\t\"Charleston County, SC\"\t45019\n\"Dorchester County, SC\"\t45035\t\"Colleton County, SC\"\t45029\n\"Dorchester County, SC\"\t45035\t\"Dorchester County, SC\"\t45035\n\"Dorchester County, SC\"\t45035\t\"Orangeburg 
